vi "generate event.vi"(9 "event":T1, 10 "queue index":i32, 11 "event queue in":T2) -> (1 "failed?":bool, 3 "event queue out":T2)   [LabVIEW 2013, in "data bus events.lvlib"]
uses:
  data bus events.lvlib
  event.ctl
  event queue element.ctl
  event queue.ctl
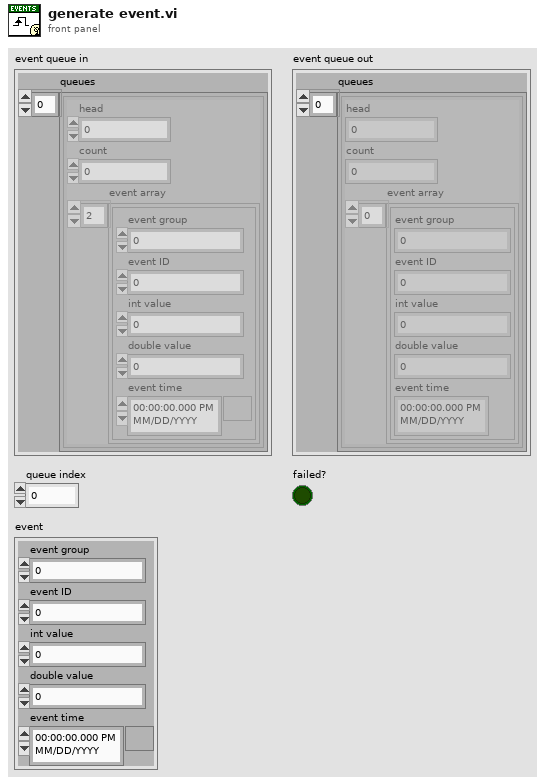
[diagram p1: front panel]
types:
  T1 = typedef "data bus events.lvlib/event.ctl" = cluster{"event group":i64, "event ID":i64, "int value":i64, "double value":dbl, "event time":timestamp}
  T2 = typedef "data bus events.lvlib/event queue.ctl" = cluster{"queues":T3[]}
  T3 = typedef "data bus events.lvlib/event queue element.ctl" = cluster{"head":i32, "count":i32, "event array":T1[]}
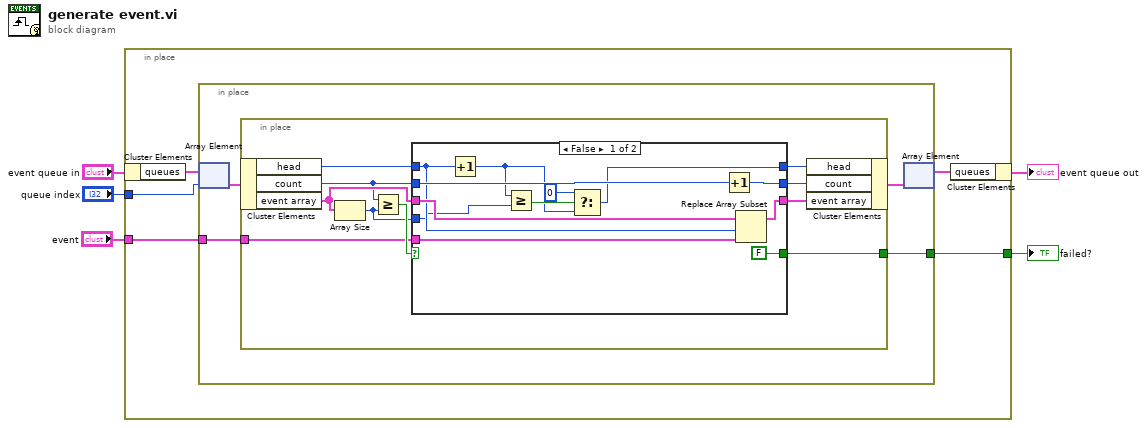
[diagram p0: block diagram]
diagram:
  n1 = in-place {
    in-place-border: "queue index" -> [w8]
    in-place-border: "event" -> [w7]
    in-place-border: [w6] -> w1
    n2 = in-place-cluster #1("event queue in") -> ("queues"=w10:T3[])
    n3 = in-place {
      in-place-border: w7 -> [w12]
      in-place-border: [w11] -> w6
      n4 = in-place-array #2(w10, w8) -> (w14:T3)
      n5 = in-place {
        in-place-border: w12 -> [w23]
        in-place-border: [w22] -> w11
        n6 = in-place-cluster #3(w14) -> ("head"=w17:i32, "count"=w20:i32, "event array"=w21:T1[])
        n7 = Array Size(array=w21) -> (size(s)=w16:i32)
        n8 = Greater Or Equal?(x=w20, y=w16) -> (x >= y?=w24:bool)
        n9 = case shown="False" w24 {
          selector: w24 -> [_ w40]
          tunnel: w23 -> [w33 _]
          tunnel: [FALSE w40] -> w22
          tunnel: w21 -> [w35 w38]
          tunnel: w20 -> [w32 w39]
          tunnel: [w31 w39] -> w19
          tunnel: [w34 w38] -> w18
          tunnel: w17 -> [w30 w37]
          tunnel: w16 -> [w28 _]
          tunnel: [w26 w37] -> w15
          frame False {
            n10 = Increment(x=w30) -> (x+1=w27:i32)
            n11 = Greater Or Equal?(x=w27, y=w28) -> (x >= y?=w29:bool)
            n12 = Select(t=0, s=w29, f=w27) -> (s? t:f=w26:i32)
            n13 = Increment(x=w32) -> (x+1=w31:i32)
            n14 = Replace Array Subset(array=w35, new element=w33, index=w30) -> (w34:T1[])
          }
          frame True {
          }
        }
        n15 = in-place-cluster #3("head"=w15, "count"=w19, "event array"=w18) -> (w13:T3)
      }
      n16 = in-place-array #2(w13) -> (w9:T3[])  [unwired: 1 out]
    }
    n17 = in-place-cluster #1("queues"=w9) -> (→"event queue out":T2)
  }
  "failed?" <- w1
